vi "Add Walk State FGV.vi"(1 "FGV Function":enum16{"Clear", "Set", "Read"}(ring)=enum."Read") -> (0 "Boolean Indicator":bool)   [LabVIEW 2012]
doc: "VI with FGV Function List Control Sub-VI and a Boolean Indicator (for use as a Functional Global Variable). \nHas properties in setting Boolean Indicator true or false for use alongside main VI:\nSet - To set Wating when the Walk button has been pressed\nRead - On the Red state, the main VI reads if Waiting is true\nClear - To clear Waiting when the Walking state begins"
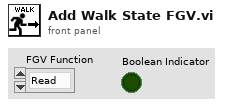
[diagram p1: front panel]
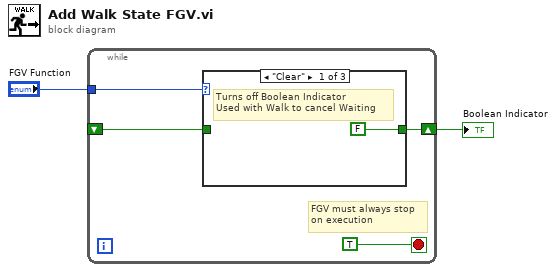
[diagram p0: block diagram]
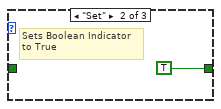
[diagram p2: hidden frame]
diagram:
  n1 = while {
    tunnel: "FGV Function" -> [w6]
    shift-right: [w4] -> w1
    shift-left: _ -> [w3]
    stop <- TRUE stop-if-true
    # "FGV must always stop\non execution"
    n2 = case shown="\"Clear\"" w6 {
      tunnel: [FALSE TRUE w9] -> w4
      tunnel: w3 -> [_ _ w9]
      frame "Clear" {
        # "Turns off Boolean Indicator\nUsed with Walk to cancel Waiting"
      }
      frame "Set" {
        # "Sets Boolean Indicator \nto True"
      }
      frame "Read" {
        # "Reads Last Boolean"
      }
    }
  }
  "Boolean Indicator" <- w1
